vi "MCCMSG Get Fast Comp Cap.vi"(8 "error in (no error)":errorcluster, 9 "pnError":i32, 10 "pdFastCompCap":dbl, 11 "hMCCmsg":i32) -> (0 "error out":errorcluster, 1 "pnError out":i32, 2 "pdFastCompCap out":dbl, 3 "function return":i32)   [LabVIEW 2012, in "MultiClamp 700B Controls.lvlib" / "AxMultiClampMsg.lvlib"]
doc: "AXMCCMSG BOOL WINAPI MCCMSG_GetFastCompCap(HMCCMSG hMCCmsg, double *pdFastCompCap, int *pnError);"
uses:
  AxMultiClampMsg.lvlib
  AxMultiClampMsg.dll
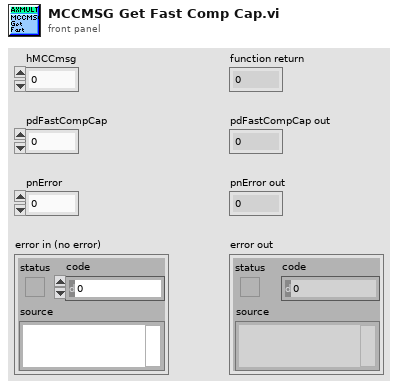
[diagram p1: front panel]
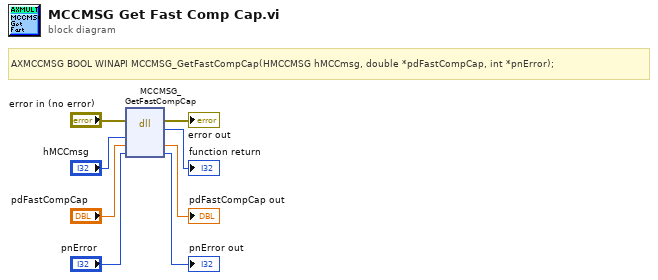
[diagram p0: block diagram]
diagram:
  # "AXMCCMSG BOOL WINAPI MCCMSG_GetFastCompCap(HMCCMSG hMCCmsg, double *pdFastCompCap, int *pnError);"
  n1 = dll-call lib="C:/Users/Southampton/Desktop/Rita/Multiclamp 700B VIs/AxMultiClampMsg/AxMultiClampMsg.*" fn="MCCMSG_GetFastCompCap"(error in="error in (no error)", "hMCCmsg"="hMCCmsg", "pdFastCompCap"="pdFastCompCap", "pnError"="pnError") -> (error out=→"error out":errorcluster, →"function return":i32, "pdFastCompCap"=→"pdFastCompCap out":dbl, "pnError"=→"pnError out":i32)  [unwired: 3 in, 1 out]
